vi "Main.vi"() -> ()   [LabVIEW 2015]
doc: "This template is for the Queued Message Handler design pattern.\n\nThe Event Handling Loop generates messages based on user interface actions.\n\nThe Message Handling Loop processes messages generated by the Event Handling Loop, or by other messages. The messages are string values, so new messages can be added easily to the Message Cases case structure in the Message Handling Loop. Each message cluster can also provide an optional value for Message Data, which is a variant that can be converted to whatever message-specific data is required."
uses:
  controls/UI Data.ctl
  support/Message Queue/Enqueue Message (Single).vi
  <vilib>/Utility/error.llb/Error Cluster From Error Code.vi
  <vilib>/ErrorRing/Error Ring.xnode
  support/Message Queue/Message Queue.lvlib
  support/User Event - Stop/User Event - Stop.lvlib
panel:
  out "Display <Replace Me> 2":string
  out "I/F type":string caption="Interface type"
  out "GB ID":string="\r\n" caption="GB Instrument ID"
  out "HP ID":string="\r\n" caption="Hi-Pot Instrument ID"
  out "Results GB":string
  out "Status GB":string
  out "Results HP":string
  out "Status HP":string
  in  "Stop GB":bool
  in  "Start GB":bool
  out "Display <Replace Me>":string
  in  "Stop Hi-Pot":bool
  in  "Start Hi-Pot":bool
  in  "Exit":bool
  # "QMH version"
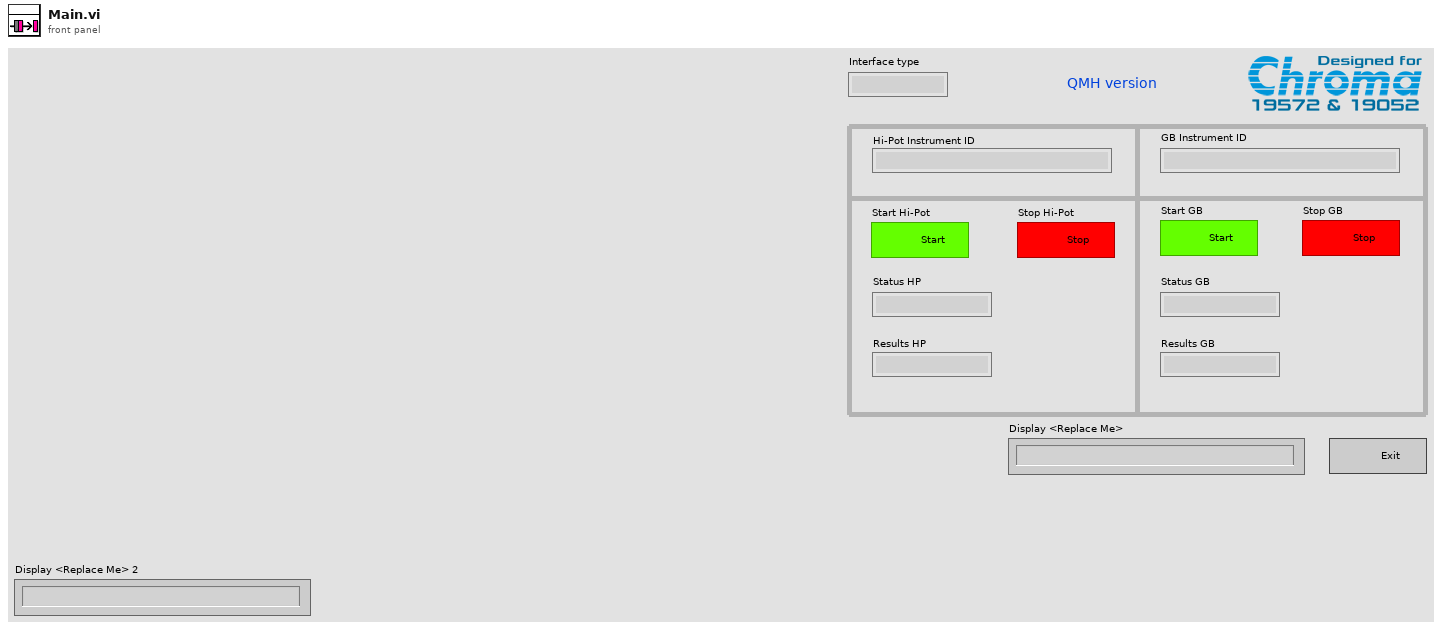
[diagram p1: front panel]
types:
  T1 = typedef "UI Data.ctl" = cluster{"Boolean <Replace Me>":bool, "Status HP":string, "Numeric <Replace Me>":dbl, "Do Something Ref":refnum<vi>, "Do Something Else Ref":refnum<vi>, "Data Display Ref":refnum<vi>, "Exit Button Ref":refnum<vi>, "Results HP":string}
  T2 = cluster{"Rsrc name for 19572":refnum<visa-resource-name>, "Rsrc name for 19052":refnum<visa-resource-name>, "I/F type":string, "VISA2 Inst ID":string, "VISA1 Inst ID":string}
  T3 = typedef "Message Queue.lvlib/All Message Queues.ctl" = cluster{"UI":refnum<queue>, "Hi-Pot Test":refnum<queue>, "GB Test":refnum<queue>}
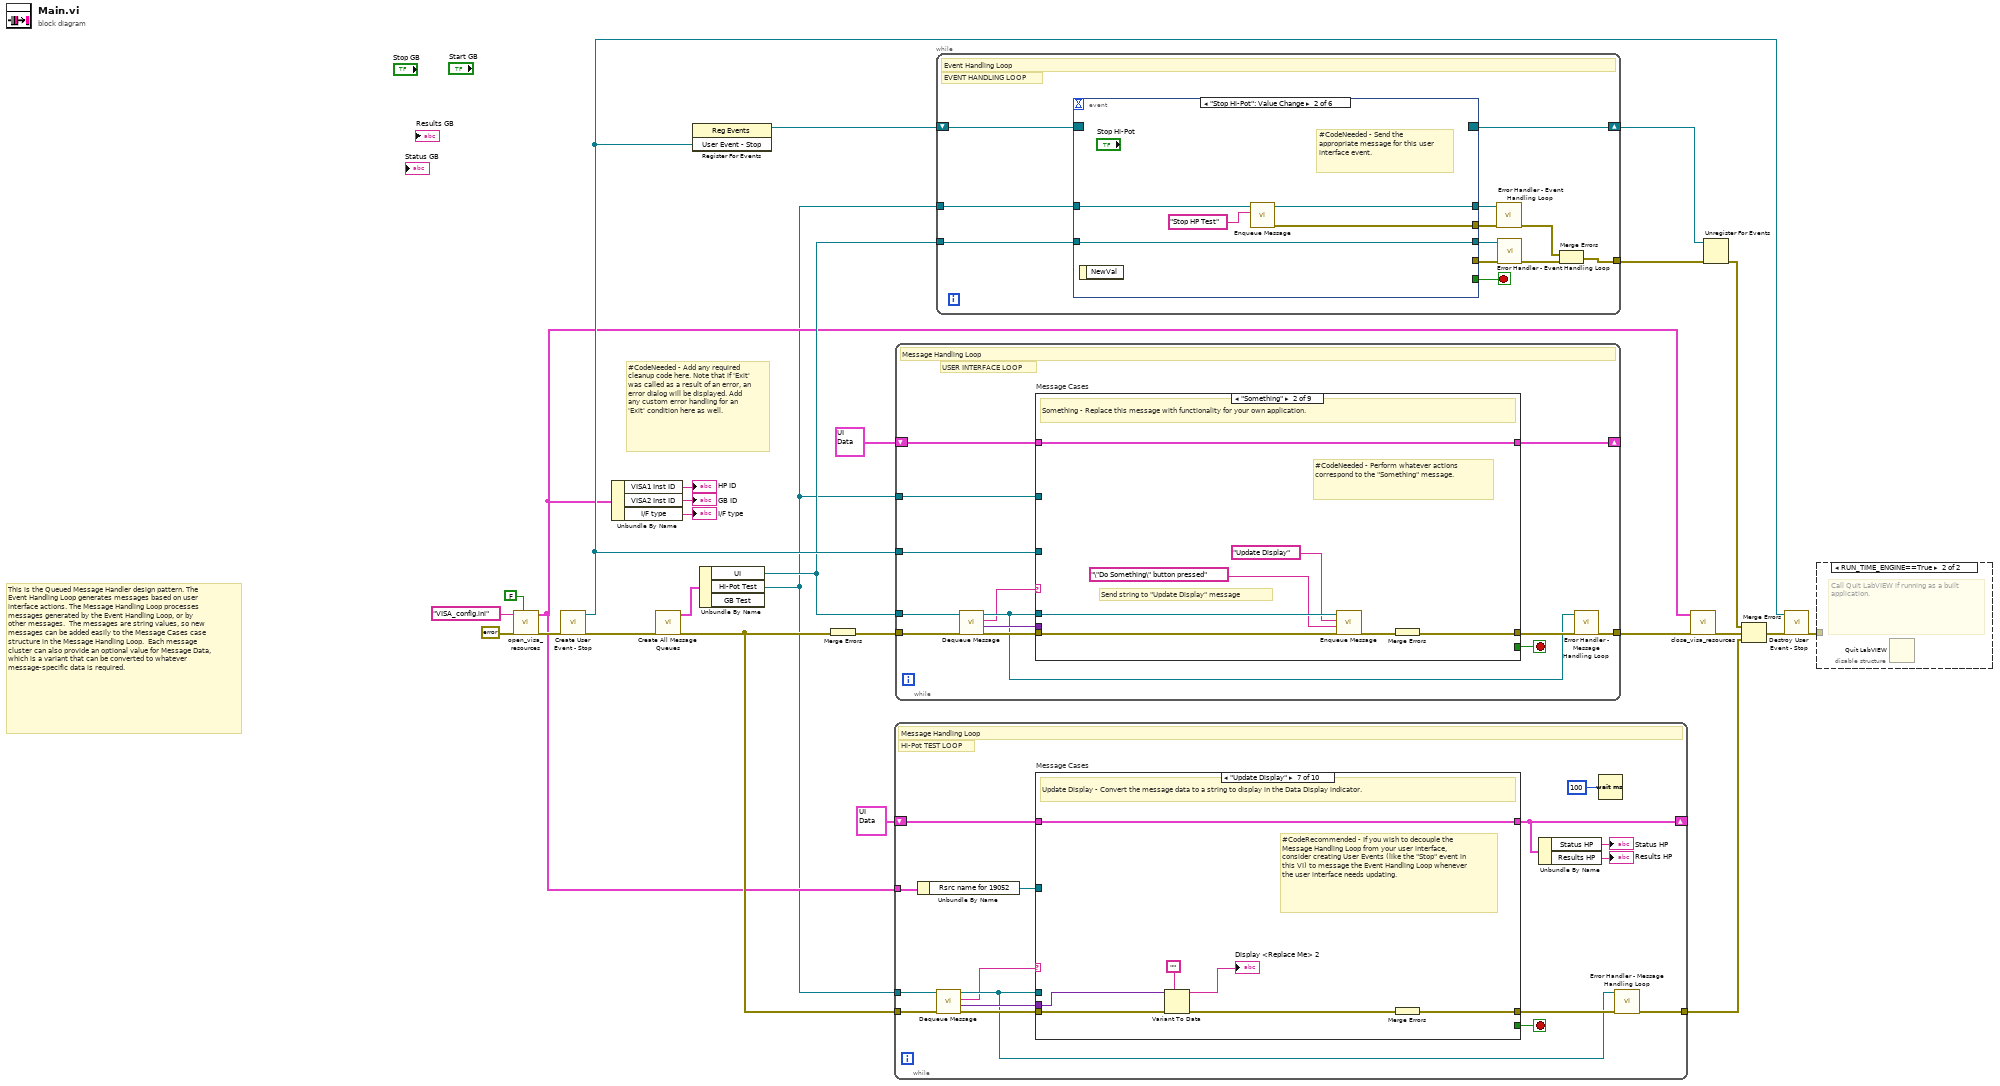
[diagram p0: block diagram]
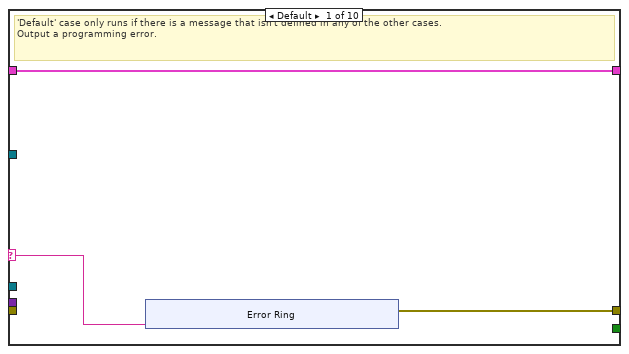
[diagram p2: hidden frame]
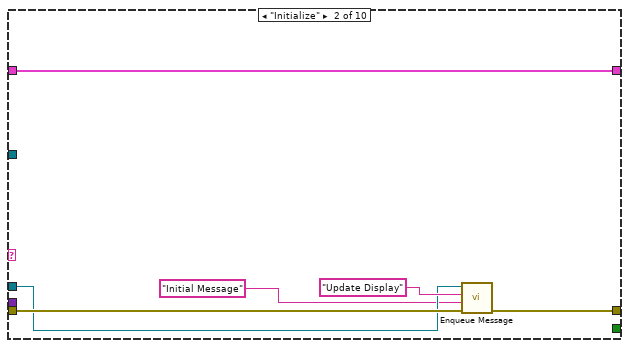
[diagram p3: hidden frame]
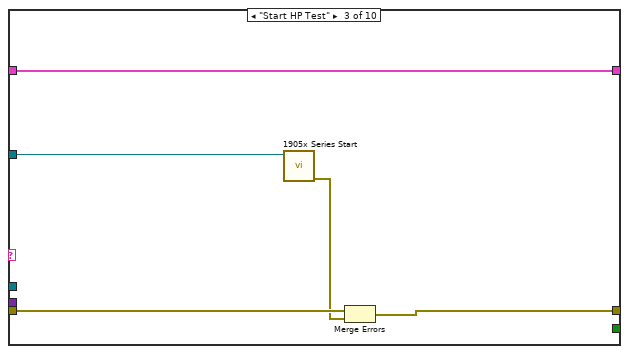
[diagram p4: hidden frame]
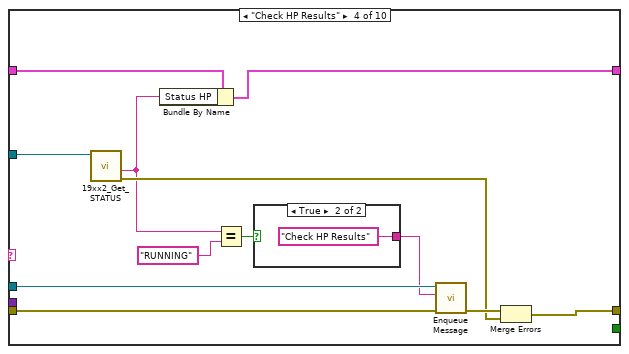
[diagram p5: hidden frame]
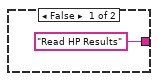
[diagram p6: hidden frame]
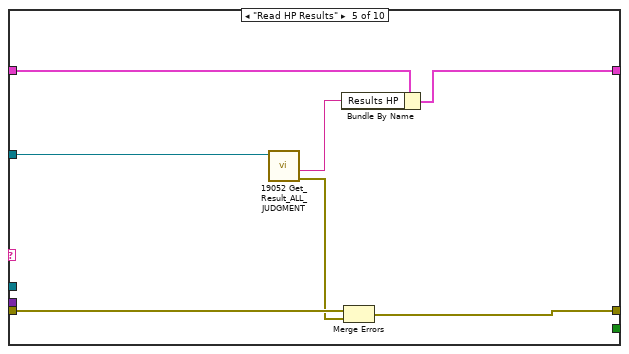
[diagram p7: hidden frame]
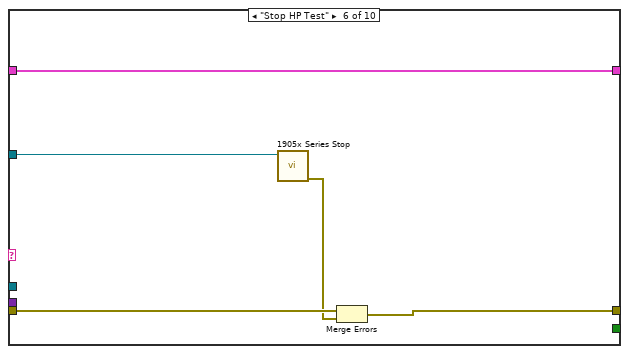
[diagram p8: hidden frame]
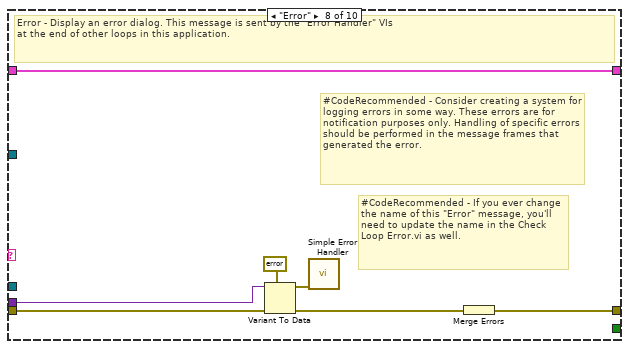
[diagram p9: hidden frame]
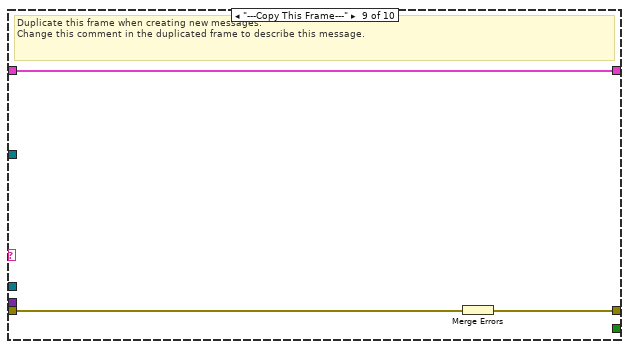
[diagram p10: hidden frame]
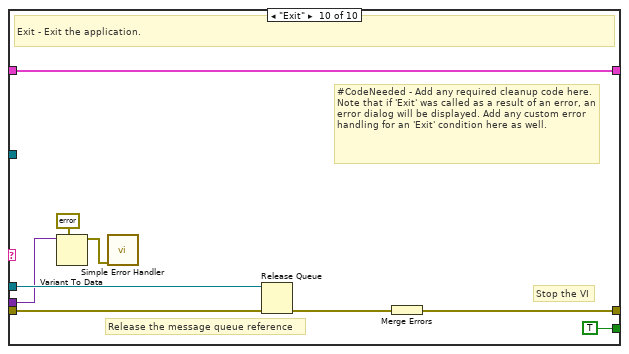
[diagram p11: hidden frame]
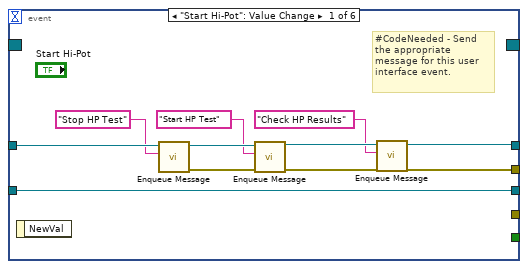
[diagram p13: hidden frame]
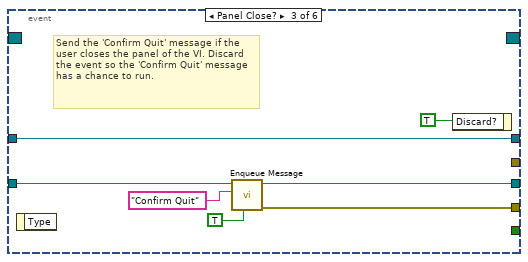
[diagram p14: hidden frame]
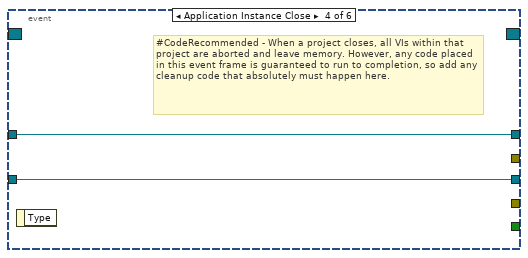
[diagram p15: hidden frame]
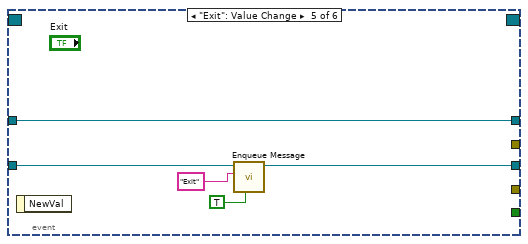
[diagram p16: hidden frame]
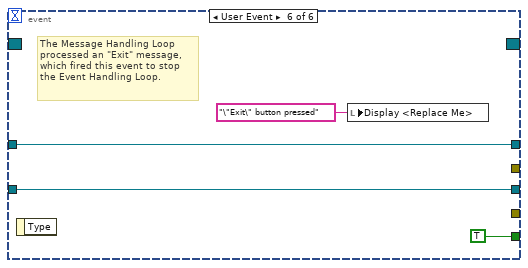
[diagram p17: hidden frame]
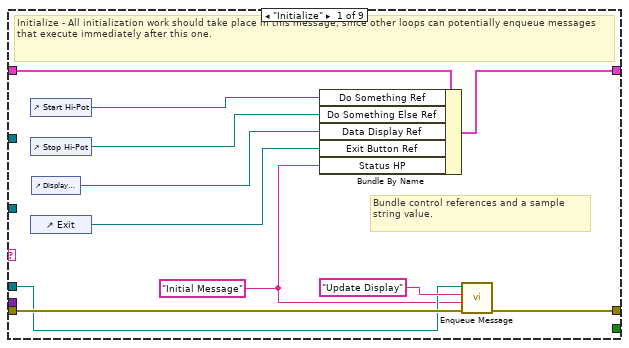
[diagram p18: hidden frame]
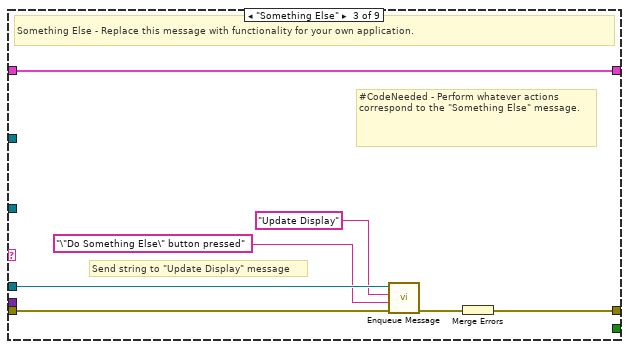
[diagram p19: hidden frame]
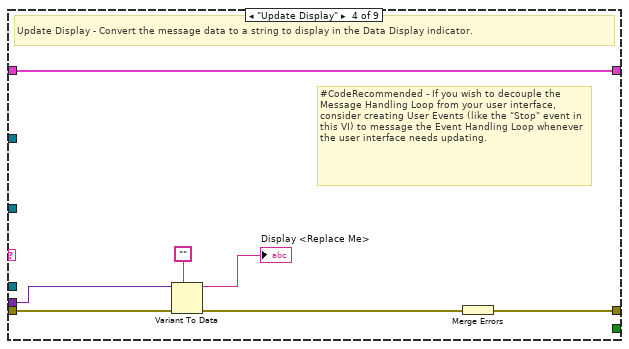
[diagram p20: hidden frame]
diagram:
  # "#CodeNeeded - Add any required cleanup code here. Note that if 'Exit' was called as a result of an error, an error dialog will be displayed. Add any custom error handling for an 'Exit' condition here as well."
  # "This is the Queued Message Handler design pattern. The Event Handling Loop generates messages based on user interface actions. The Message Handling Loop processes messages generated by the Event Handling Loop, or by other messages.  The messages are string values, so new messages can be added easily to the Message Cases case structure in the Message Handling Loop.  Each message cluster can also provide an optional value for Message Data, which is a variant that can be converted to whatever message-specific data is required."
  n1 = call "open_visa_resources.vi"("test mode"=FALSE, "error in (no error)"=errorcluster {"status"=FALSE, "code"=0, "source"=""} ("error constant"), "config file in"="VISA_config.ini") -> ("error out"=w5:errorcluster, "VISA out"=w2:T2)  [unwired: 7 in]
  n2 = call "Create User Event - Stop.vi"("error in (no error)"=w5) -> ("error out"=w25:errorcluster, "User Event - Stop"=w17:refnum<user-event>)  [unwired: 9 in]
  n3 = Unbundle By Name(w2) -> ("VISA1 Inst ID"=→"HP ID":string, "VISA2 Inst ID"=→"GB ID":string, "I/F type"=→"I/F type":string)
  n4 = call "Create All Message Queues.vi"("error in (no error)"=w25) -> ("error out"=w26:errorcluster, "Message Queues out"=w16:T3)  [unwired: 9 in]
  n5 = register-events(w17) -> (reference out=w18:refnum<event-registration>)  [unwired: 2 in, 1 out]
  n6 = Unbundle By Name(w16) -> ("UI"=w15:refnum<queue>, "Hi-Pot Test"=w1:refnum<queue>)  [unwired: 1 out]
  n7 = Merge Errors(w26) -> (w6:errorcluster)
  n8 = while {
    tunnel: w1 -> [w37]
    shift-right: [w30] -> _
    shift-left: T1 {"Boolean <Replace Me>"=FALSE, "Status HP"="", "Numeric <Replace Me>"=0.0, "Do Something Ref"=refnum, "Do Something Else Ref"=refnum, "Data Display Ref"=refnum, "Exit Button Ref"=refnum, "Results HP"=""} ("Data Cluster") -> [w41]
    tunnel: w26 -> [w40]
    tunnel: [w35] -> w14
    tunnel: w2 -> [w32]
    stop <- w34 stop-if-true
    # "Hi-Pot TEST LOOP"
    # "Message Handling Loop"
    n9 = Unbundle By Name(w32) -> ("Rsrc name for 19052"=w31:refnum<visa-resource-name>)
    n10 = call "Dequeue Message.vi"("error in (no error)"=w40, "Message Queue"=w37) -> ("error out"=w39:errorcluster, "Message Data"=w38:variant, "Message"=w33:string, "dup Message Queue"=w36:refnum<queue>)  [unwired: 6 in]
    n11 = case "Message Cases" shown="\"Update Display\"" w33 {
      selector: w33 -> [w43 _ _ _ _ _ _ _ _ _]
      tunnel: w36 -> [_ w55 _ w72 _ _ _ _ _ w115]
      tunnel: w39 -> [_ w57 w61 w74 w84 w86 w94 w103 w106 w110]
      tunnel: [w44 w58 w60 w75 w83 w88 w95 w97 w104 w111] -> w42
      tunnel: w41 -> [w45 w53 w63 w70 w80 w89 w96 w102 w105 w114]
      tunnel: [w45 w53 w63 w69 w79 w89 w96 w102 w105 w114] -> w30
      tunnel: [_ _ _ _ _ _ _ _ _ TRUE] -> w34
      tunnel: w38 -> [_ _ _ _ _ _ w93 w101 _ w107]
      tunnel: w31 -> [_ _ w62 w71 w82 w87 _ _ _ _]
      frame Default {
        # "'Default' case only runs if there is a message that isn't defined in any of the other cases. \nOutput a programming error."
        n12 = xnode "Error Ring"("parameter 0"=w43) -> ("error out"=w44:errorcluster)
      }
      frame "Initialize" {
        n13 = call-poly "Enqueue Message.vi"("error in (no error)"=w57, "Message Data"="Initial Message" ("Initial Message"), "Message"="Update Display", "Message Queue"=w55) -> ("error out"=w58:errorcluster)  [unwired: 6 in, 1 out]
      }
      frame "Start HP Test" {
        n14 = call "1905x Series Start.vi"("VISA resource in"=w62) -> ("error out"=w59:errorcluster)  [unwired: 9 in, 1 out]
        n15 = Merge Errors(w61, w59) -> (w60:errorcluster)
      }
      frame "Check HP Results" {
        n16 = call "19xx2_Get_STATUS.vi"("VISA resource in"=w71) -> ("error out"=w65:errorcluster, "Status"=w64:string)  [unwired: 8 in, 1 out]
        n17 = Bundle By Name(cluster=w70, "Status HP"=w64) -> (w69:T1)
        n18 = Equal?(x=w64, y="RUNNING") -> (x = y?=w67:bool)
        n19 = case shown="True" w67 {
          tunnel: ["Read HP Results" ("program string") "Check HP Results" ("Message")] -> w66
          frame False {
          }
          frame True {
          }
        }
        n20 = call-poly "Enqueue Message.vi"("error in (no error)"=w74, "Message"=w66, "Message Queue"=w72) -> ("error out"=w73:errorcluster)  [unwired: 7 in, 1 out]
        n21 = Merge Errors(w73, w65) -> (w75:errorcluster)
      }
      frame "Read HP Results" {
        n22 = call "19052 Get_Result_ALL_JUDGMENT.vi"("VISA resource in"=w82) -> ("error out"=w81:errorcluster, "JUDGMENT"=w78:string)  [unwired: 8 in, 1 out]
        n23 = Bundle By Name(cluster=w80, "Results HP"=w78) -> (w79:T1)
        n24 = Merge Errors(w84, w81) -> (w83:errorcluster)
      }
      frame "Stop HP Test" {
        n25 = call "1905x Series Stop.vi"("VISA resource in"=w87) -> ("error out"=w85:errorcluster)  [unwired: 9 in, 1 out]
        n26 = Merge Errors(w86, w85) -> (w88:errorcluster)
      }
      frame "Update Display" {
        # "#CodeRecommended - If you wish to decouple the Message Handling Loop from your user interface, consider creating User Events (like the \"Stop\" event in this VI) to message the Event Handling Loop whenever the user interface needs updating."
        # "Update Display - Convert the message data to a string to display in the Data Display indicator."
        n27 = Variant To Data(error in=w94, type="", Variant=w93) -> (data=→"Display <Replace Me> 2":string, error out=w91:errorcluster)
        n28 = Merge Errors(w91) -> (w95:errorcluster)
      }
      frame "Error" {
        # "#CodeRecommended - If you ever change the name of this \"Error\" message, you'll need to update the name in the Check Loop Error.vi as well."
        # "#CodeRecommended - Consider creating a system for logging errors in some way. These errors are for notification purposes only. Handling of specific errors should be performed in the message frames that generated the error."
        # "Error - Display an error dialog. This message is sent by the \"Error Handler\" VIs \nat the end of other loops in this application."
        n29 = Variant To Data(error in=w103, type=errorcluster {"status"=FALSE, "code"=0, "source"=""} ("error constant"), Variant=w101) -> (data=w99:errorcluster, error out=w98:errorcluster)
        n30 = call <vilib>:"Simple Error Handler.vi"("error in (no error)"=w99) -> ()  [unwired: 4 in, 5 out]
        n31 = Merge Errors(w98) -> (w97:errorcluster)
      }
      frame "---Copy This Frame---" {
        # "Duplicate this frame when creating new messages.\nChange this comment in the duplicated frame to describe this message."
        n32 = Merge Errors(w106) -> (w104:errorcluster)
      }
      frame "Exit" {
        # "Stop the VI"
        # "Release the message queue reference"
        # "#CodeNeeded - Add any required cleanup code here. Note that if 'Exit' was called as a result of an error, an error dialog will be displayed. Add any custom error handling for an 'Exit' condition here as well."
        # "Exit - Exit the application."
        n33 = Variant To Data(type=errorcluster {"status"=FALSE, "code"=0, "source"=""} ("error constant"), Variant=w107) -> (data=w108:errorcluster)  [unwired: 1 in, 1 out]
        n34 = call <vilib>:"Simple Error Handler.vi"("error in (no error)"=w108) -> ()  [unwired: 4 in, 5 out]
        n35 = Release Queue(queue=w115, error in (no error)=w110) -> (error out=w112:errorcluster)  [unwired: 1 in, 2 out]
        n36 = Merge Errors(w112) -> (w111:errorcluster)
      }
    }
    n37 = Unbundle By Name(w30) -> ("Status HP"=→"Status HP":string, "Results HP"=→"Results HP":string)
    n38 = Wait (ms)(milliseconds to wait=u32 100) -> ()  [unwired: 1 out]
    n39 = call "Error Handler - Message Handling Loop.vi"("error in (no error)"=w42, "Message Queue"=w36) -> ("dup error in"=w35:errorcluster)  [unwired: 8 in, 1 out]
  }
  n40 = while {
    tunnel: w15 -> [w121]
    shift-right: [w126] -> _
    shift-left: T1 {"Boolean <Replace Me>"=FALSE, "Status HP"="", "Numeric <Replace Me>"=0.0, "Do Something Ref"=refnum, "Do Something Else Ref"=refnum, "Data Display Ref"=refnum, "Exit Button Ref"=refnum, "Results HP"=""} ("Data Cluster") -> [w127]
    tunnel: w17 -> [w125]
    tunnel: w6 -> [w124]
    tunnel: [w119] -> w4
    tunnel: w1 -> [w116]
    stop <- w118 stop-if-true
    # "USER INTERFACE LOOP"
    # "Message Handling Loop"
    n41 = call "Dequeue Message.vi"("error in (no error)"=w124, "Message Queue"=w121) -> ("error out"=w123:errorcluster, "Message Data"=w122:variant, "Message"=w117:string, "dup Message Queue"=w120:refnum<queue>)  [unwired: 6 in]
    n42 = case "Message Cases" shown="\"Something\"" w117 {
      selector: w117 -> [_ _ _ _ _ _ _ _ w193]
      tunnel: w120 -> [w130 w142 w149 _ _ w170 _ w192 _]
      tunnel: w123 -> [w138 w144 w151 w158 w167 w174 w177 w187 _]
      tunnel: [w139 w145 w152 w159 w161 w172 w175 w189 w194] -> w128
      tunnel: w127 -> [w137 w146 w153 w160 w166 w173 w176 w191 w195]
      tunnel: [w136 w146 w153 w160 w166 w173 w176 w191 w195] -> w126
      tunnel: [_ _ _ _ _ _ _ TRUE _] -> w118
      tunnel: w122 -> [_ _ _ w157 w165 _ _ w184 _]
      tunnel: w125 -> [_ _ _ _ _ _ _ w188 _]
      tunnel: w116 -> [_ _ _ _ _ _ _ w182 _]
      frame "Initialize" {
        w129 = "Initial Message" ("Initial Message")
        # "Bundle control references and a sample string value."
        # "Initialize - All initialization work should take place in this message, since other loops can potentially enqueue messages that execute immediately after this one."
        n43 = control-ref of="Start Hi-Pot"() -> (w135:refnum<vi>)
        n44 = control-ref of="Stop Hi-Pot"() -> (w134:refnum<vi>)
        n45 = control-ref of="Exit"() -> (w132:refnum<vi>)
        n46 = control-ref of="Display <Replace Me>"() -> (w133:refnum<vi>)
        n47 = Bundle By Name(cluster=w137, "Do Something Ref"=w135, "Do Something Else Ref"=w134, "Data Display Ref"=w133, "Exit Button Ref"=w132, "Status HP"=w129) -> (w136:T1)
        n48 = call-poly "Enqueue Message.vi"("error in (no error)"=w138, "Message Data"=w129, "Message"="Update Display", "Message Queue"=w130) -> ("error out"=w139:errorcluster)  [unwired: 6 in, 1 out]
      }
      frame "Something" {
        # "Send string to \"Update Display\" message"
        # "#CodeNeeded - Perform whatever actions correspond to the \"Something\" message."
        # "Something - Replace this message with functionality for your own application."
        n49 = call-poly "Enqueue Message.vi"("error in (no error)"=w144, "Message Data"="\"Do Something\" button pressed" ("\"Do Something\" button pressed"), "Message"="Update Display", "Message Queue"=w142) -> ("error out"=w143:errorcluster)  [unwired: 6 in, 1 out]
        n50 = Merge Errors(w143) -> (w145:errorcluster)
      }
      frame "Something Else" {
        # "Send string to \"Update Display\" message"
        # "#CodeNeeded - Perform whatever actions correspond to the \"Something Else\" message."
        # "Something Else - Replace this message with functionality for your own application."
        n51 = call-poly "Enqueue Message.vi"("error in (no error)"=w151, "Message Data"="\"Do Something Else\" button pressed" ("\"Do Something Else\" button pressed"), "Message"="Update Display", "Message Queue"=w149) -> ("error out"=w150:errorcluster)  [unwired: 6 in, 1 out]
        n52 = Merge Errors(w150) -> (w152:errorcluster)
      }
      frame "Update Display" {
        # "#CodeRecommended - If you wish to decouple the Message Handling Loop from your user interface, consider creating User Events (like the \"Stop\" event in this VI) to message the Event Handling Loop whenever the user interface needs updating."
        # "Update Display - Convert the message data to a string to display in the Data Display indicator."
        n53 = Variant To Data(error in=w158, type="", Variant=w157) -> (data=→"Display <Replace Me>":string, error out=w155:errorcluster)
        n54 = Merge Errors(w155) -> (w159:errorcluster)
      }
      frame "Error" {
        # "#CodeRecommended - If you ever change the name of this \"Error\" message, you'll need to update the name in the Check Loop Error.vi as well."
        # "#CodeRecommended - Consider creating a system for logging errors in some way. These errors are for notification purposes only. Handling of specific errors should be performed in the message frames that generated the error."
        # "Error - Display an error dialog. This message is sent by the \"Error Handler\" VIs \nat the end of other loops in this application."
        n55 = Variant To Data(error in=w167, type=errorcluster {"status"=FALSE, "code"=0, "source"=""} ("error constant"), Variant=w165) -> (data=w163:errorcluster, error out=w162:errorcluster)
        n56 = call <vilib>:"Simple Error Handler.vi"("error in (no error)"=w163) -> ()  [unwired: 4 in, 5 out]
        n57 = Merge Errors(w162) -> (w161:errorcluster)
      }
      frame "Confirm Quit" {
        # "#CodeNeeded - If you want to provide an \"Are you sure\" dialog (or some other notification) before the application exits, place that code here. This message is typically sent from a Panel Close? event."
        # "Confirm Quit - Message that can confirm whether or not the user wants to exit the application."
        n58 = call-poly "Enqueue Message.vi"("Priority Message? (F)"=TRUE, "error in (no error)"=w174, "Message"="Exit", "Message Queue"=w170) -> ("error out"=w171:errorcluster)  [unwired: 6 in, 1 out]
        n59 = Merge Errors(w171) -> (w172:errorcluster)
      }
      frame "---Copy This Frame---" {
        # "Duplicate this frame when creating new messages.\nChange this comment in the duplicated frame to describe this message."
        n60 = Merge Errors(w177) -> (w175:errorcluster)
      }
      frame "Exit" {
        # "Stop the VI"
        # "Release the message queue reference"
        # "Exit - Exit the application."
        n61 = Variant To Data(type=errorcluster {"status"=FALSE, "code"=0, "source"=""} ("error constant"), Variant=w184) -> (data=w185:errorcluster)  [unwired: 1 in, 1 out]
        n62 = call <vilib>:"Simple Error Handler.vi"("error in (no error)"=w185) -> ()  [unwired: 4 in, 5 out]
        n63 = call-poly "Enqueue Message.vi"("Priority Message? (F)"=TRUE, "Message"="Exit", "Message Queue"=w182) -> ("error out"=w179:errorcluster)  [unwired: 7 in, 1 out]
        n64 = call "Fire User Event - Stop.vi"("User Event - Stop"=w188) -> ("error out"=w178:errorcluster)  [unwired: 10 in]
        n65 = Release Queue(queue=w192, error in (no error)=w187) -> (error out=w180:errorcluster)  [unwired: 1 in, 2 out]
        n66 = Merge Errors(w180, w179, w178) -> (w189:errorcluster)
      }
      frame Default {
        # "'Default' case only runs if there is a message that isn't defined in any of the other cases. \nOutput a programming error."
        n67 = xnode "Error Ring"("parameter 0"=w193) -> ("error out"=w194:errorcluster)
      }
    }
    n68 = call "Error Handler - Message Handling Loop.vi"("error in (no error)"=w128, "Message Queue"=w120) -> ("dup error in"=w119:errorcluster)  [unwired: 8 in, 1 out]
  }
  n69 = while {
    tunnel: w15 -> [w214]
    shift-right: [w212] -> w22
    shift-left: w18 -> [w213]
    tunnel: [w204] -> w19
    tunnel: w1 -> [w207]
    stop <- w210 stop-if-true
    # "EVENT HANDLING LOOP"
    # "Event Handling Loop"
    n70 = event shown="[1] \"Stop Hi-Pot\": Value Change" {
      selector: w213 -> [_ _ _ _ _ _]
      dyn-events: [_ _ _ _ _ _] -> w212
      timeout: _ -> [_ _ _ _ _ _]
      tunnel: [_ _ _ _ _ TRUE ("Discard?")] -> w210
      tunnel: w214 -> [w222 w228 w235 w238 w240 w247]
      tunnel: [_ _ w234 _ _ _] -> w211
      tunnel: [w222 w228 w233 w238 w239 w247] -> w209
      tunnel: w207 -> [w224 w227 w230 w237 w243 w244]
      tunnel: [w216 w226 w230 w237 w243 w244] -> w206
      tunnel: [w219 w225 _ _ _ _] -> w205
      event "Start Hi-Pot": Value Change {
        # "#CodeNeeded - Send the appropriate message for this user interface event."
        n71 = event-data() -> ()  [unwired: 1 in, 1 out]
        n72 = call-poly "Enqueue Message.vi"("Message"="Stop HP Test", "Message Queue"=w224) -> ("error out"=w220:errorcluster, "dup Message Queue"=w221:refnum<queue>)  [unwired: 8 in]
        n73 = call-poly "Enqueue Message.vi"("error in (no error)"=w220, "Message"="Start HP Test", "Message Queue"=w221) -> ("error out"=w219:errorcluster, "dup Message Queue"=w217:refnum<queue>)  [unwired: 7 in]
        n74 = call-poly "Enqueue Message.vi"("Message"="Check HP Results", "Message Queue"=w217) -> ("dup Message Queue"=w216:refnum<queue>)  [unwired: 8 in, 1 out]
      }
      event "Stop Hi-Pot": Value Change {
        # "#CodeNeeded - Send the appropriate message for this user interface event."
        n75 = event-data() -> ()  [unwired: 1 in, 1 out]
        n76 = call-poly "Enqueue Message.vi"("Message"="Stop HP Test", "Message Queue"=w227) -> ("error out"=w225:errorcluster, "dup Message Queue"=w226:refnum<queue>)  [unwired: 8 in]
      }
      event Panel Close? {
        # "Send the 'Confirm Quit' message if the user closes the panel of the VI. Discard the event so the 'Confirm Quit' message has a chance to run."
        n77 = event-data() -> ()  [unwired: 1 in, 1 out]
        n78 = call-poly "Enqueue Message.vi"("Priority Message? (F)"=TRUE, "Message"="Confirm Quit", "Message Queue"=w235) -> ("error out"=w234:errorcluster, "dup Message Queue"=w233:refnum<queue>)  [unwired: 7 in]
        n79 = event-data("Discard?"=TRUE) -> ()  [unwired: 1 in, 1 out]
      }
      event Application Instance Close {
        # "#CodeRecommended - When a project closes, all VIs within that project are aborted and leave memory. However, any code placed in this event frame is guaranteed to run to completion, so add any cleanup code that absolutely must happen here."
        n80 = event-data() -> ()  [unwired: 1 in, 1 out]
      }
      event "Exit": Value Change {
        n81 = event-data() -> ()  [unwired: 1 in, 1 out]
        n82 = call-poly "Enqueue Message.vi"("Priority Message? (F)"=TRUE, "Message"="Exit", "Message Queue"=w240) -> ("dup Message Queue"=w239:refnum<queue>)  [unwired: 7 in, 1 out]
      }
      event User Event {
        # "The Message Handling Loop processed an \"Exit\" message, which fired this event to stop the Event Handling Loop."
        n83 = event-data() -> ()  [unwired: 1 in, 1 out]
        n84 = local write "Display <Replace Me>"("\"Exit\" button pressed" ("VI Stopped")) -> ()
      }
    }
    n85 = call "Error Handler - Event Handling Loop.vi"("error in (no error)"=w205, "Message Queue"=w206) -> ("dup error in"=w203:errorcluster)  [unwired: 8 in, 1 out]
    n86 = call "Error Handler - Event Handling Loop.vi"("error in (no error)"=w211, "Message Queue"=w209) -> ("dup error in"=w208:errorcluster)  [unwired: 8 in, 1 out]
    n87 = Merge Errors(w203, w208) -> (w204:errorcluster)
  }
  n88 = call "close_visa_resources.vi"("error in (no error)"=w4, "VISA in"=w2) -> ("error out"=w3:errorcluster)  [unwired: 9 in]
  n89 = Unregister For Events(event registration refnum=w22, error in=w19) -> (error out=w23:errorcluster)
  n90 = Merge Errors(w23, w3, w14) -> (w24:errorcluster)
  n91 = call "Destroy User Event - Stop.vi"("error in (no error)"=w24, "User Event - Stop"=w17) -> ("error out"=w20:errorcluster)  [unwired: 9 in]
  n92 = disable-structure shown="RUN_TIME_ENGINE==True" {
    disable-tunnel: w20 -> [_ _]
    frame condition #0 (active) {
    }
    frame condition #1 {
      # "Call Quit LabVIEW if running as a built application."
      n93 = Quit LabVIEW() -> ()  [unwired: 1 in]
    }
  }
